vi "Do.vi"(8 "error in (no error)":errorcluster, 10 "Actor in":refnum<class "Actor.lvclass">, 11 "New Image Threshold Msg":refnum<class "New Image Threshold Msg.lvclass">) -> (0 "error out":errorcluster, 2 "Actor out":refnum<class "Actor.lvclass">)   [LabVIEW 2016, in "Tests.lvlib" / "New Image Threshold Msg.lvclass"]
doc: "This VI delivers the message to the actor by calling the appropriate method(s) on the actor."
uses:
  New Image Threshold Msg.lvclass
  C:/Users/Achu/Desktop/2015/Image Acquisition/Image Acquisition Messages/Image Msg/Image Msg.lvclass
  <vilib>/ActorFramework/Actor/Actor.lvclass
  Threshold/Threshold.lvclass
  C:/Program Files (x86)/National Instruments/LabVIEW 2016/vi.lib/ActorFramework/Actor/Actor.lvclass
  Image Acquisition/Image Acquisition Messages/Image Msg/Image Msg.lvclass/Image Msg.ctl
  Image Acquisition/Image Acquisition Messages/Image Msg/Image Msg.lvclass
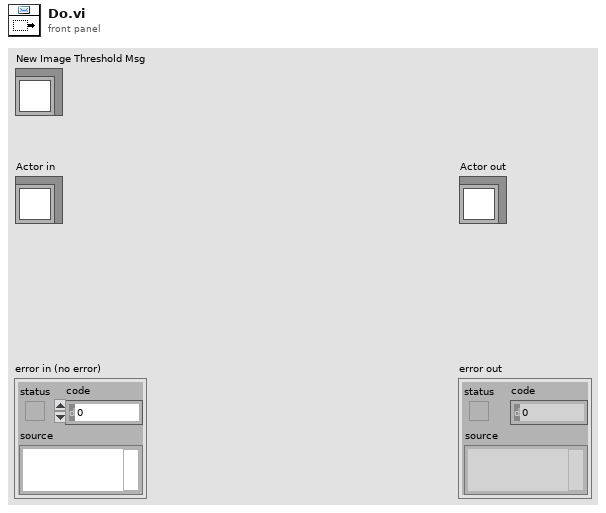
[diagram p1: front panel]
types:
  T1 = typedef "IMAQ Image.ctl" = refnum<image>
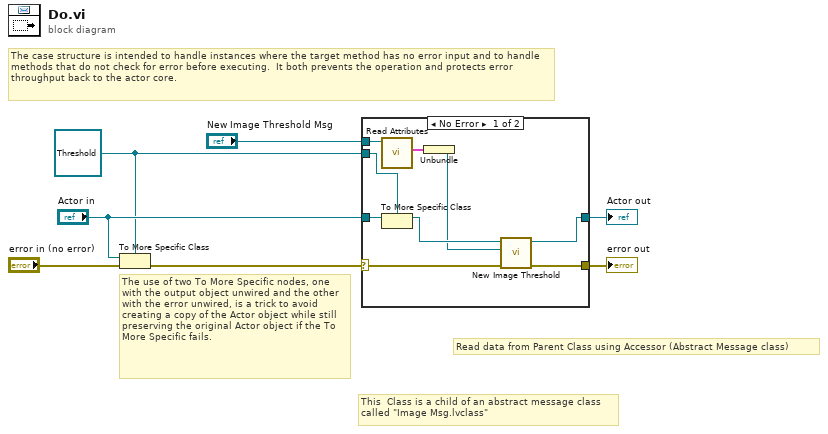
[diagram p0: block diagram]
diagram:
  w2 = refnum<class "Threshold.lvclass"> refnum ("Actor in")
  # "This  Class is a child of an abstract message class\ncalled \"Image Msg.lvclass\""
  # "Read data from Parent Class using Accessor (Abstract Message class)"
  # "The use of two To More Specific nodes, one with the output object unwired and the other with the error unwired, is a trick to avoid creating a copy of the Actor object while still preserving the original Actor object if the To More Specific fails."
  # "The case structure is intended to handle instances where the target method has no error input and to handle methods that do not check for error before executing.  It both prevents the operation and protects error throughput back to the actor core."
  n1 = To More Specific Class(target class=w2, reference="Actor in", error in="error in (no error)") -> (error out=w6:errorcluster)  [unwired: 1 out]
  n2 = case shown="No Error" w6 {
    selector: w6 -> [w14 w18]
    tunnel: [w16 w18] -> w5
    tunnel: [w15 w17] -> w4
    tunnel: "Actor in" -> [w13 w17]
    tunnel: w2 -> [w12 _]
    tunnel: "New Image Threshold Msg" -> [w9 _]
    frame No Error {
      n3 = call "Read Attributes.vi"("Image Msg"=w9) -> ("Payload"=w10:cluster{"Image":T1})  [unwired: 10 in]
      n4 = To More Specific Class(target class=w12, reference=w13) -> (specific class reference=w11:refnum<class "Threshold.lvclass">)  [unwired: 1 in, 1 out]
      n5 = Unbundle(w10) -> ("Image"=w8:T1)
      n6 = call "New Image Threshold.vi"("error in (no error)"=w14, "New Image"=w8, "Threshold in"=w11) -> ("error out"=w16:errorcluster, "Threshold out"=w15:refnum<class "Threshold.lvclass">)  [unwired: 7 in]
    }
    frame Error {
      # "If type check fails, pass the original object out again."
    }
  }
  "error out" <- w5
  "Actor out" <- w4
